vi "Send_Duration(SubVI).vi"(9 "error in (no error)":errorcluster, 10 "VISA resource name":refnum<visa-resource-name>, 11 "Set High1 Time":i16) -> (0 "error out":errorcluster, 1 "ASCII string":string[](array[string]), 2 "High1 Time(ns)":dbl, 3 "Digital Outputs":bool[](array[boolean]), 5 "VISA resource name out":refnum<visa-resource-name>, 8 "In Range?":bool)   [LabVIEW 2022 SP3]
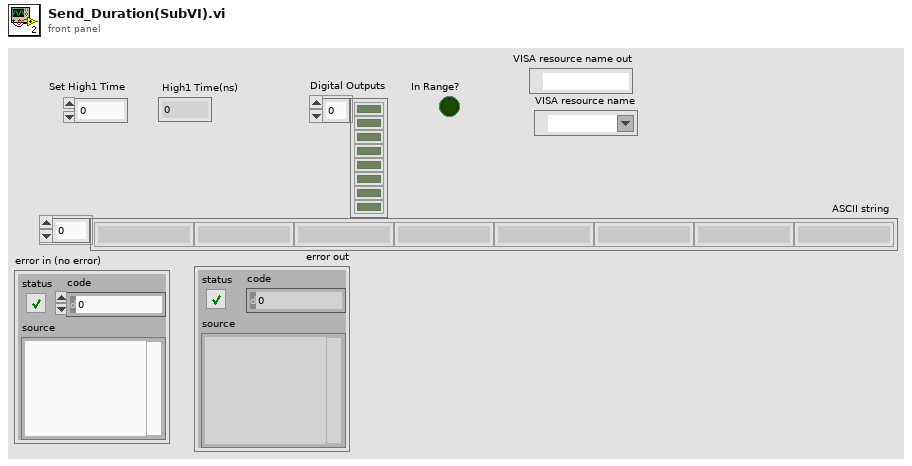
[diagram p1: front panel]
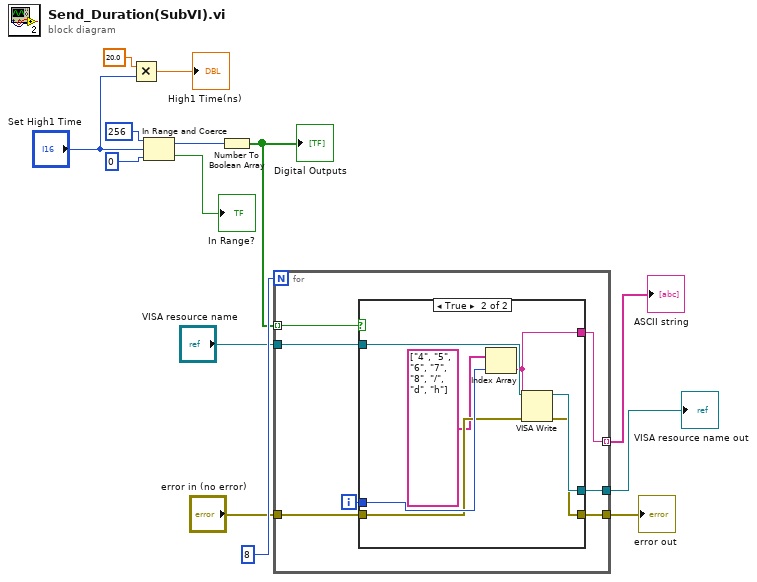
[diagram p0: block diagram]
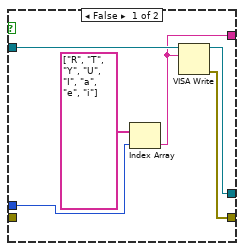
[diagram p2: hidden frame]
diagram:
  n1 = Multiply(x=20.0, y="Set High1 Time") -> (x*y=→"High1 Time(ns)":dbl)
  n2 = In Range and Coerce(upper limit=i16 256, x="Set High1 Time", lower limit=i8 0) -> (coerced(x)=w8:i16, In Range?=→"In Range?":bool)
  n3 = Number To Boolean Array(number=w8) -> (Boolean array=w9:bool[])
  "Digital Outputs" <- w9
  n4 = for {
    N: 8 -> [_]
    tunnel: w9 -> [w21] mode=indexing
    tunnel: [w19] -> w11 mode=indexing
    tunnel: "VISA resource name" -> [w18]
    tunnel: [w17] -> w3
    tunnel: [w16] -> w2
    tunnel: "error in (no error)" -> [w15]
    i -> [w20]
    n5 = case shown="True" w21 {
      tunnel: w20 -> [w27 w34]
      tunnel: [w25 w32] -> w19
      tunnel: w18 -> [w26 w33]
      tunnel: [w24 w31] -> w17
      tunnel: [w23 w30] -> w16
      tunnel: w15 -> [_ w29]
      frame False {
        n6 = Index Array(array=string[] ["R", "T", "Y", "U", "I", "a", "e", "i"] ("ASCII LOW"), index=w27) -> (element=w25:string)
        n7 = VISA Write(VISA resource name=w26, write buffer=w25) -> (VISA resource name out=w24:refnum<visa-resource-name>, error out=w23:errorcluster)  [unwired: 1 in, 1 out]
      }
      frame True {
        n8 = Index Array(array=string[] ["4", "5", "6", "7", "8", "/", "d", "h"] ("ASCII HIGH"), index=w34) -> (element=w32:string)
        n9 = VISA Write(VISA resource name=w33, write buffer=w32, error in (no error)=w29) -> (VISA resource name out=w31:refnum<visa-resource-name>, error out=w30:errorcluster)  [unwired: 1 out]
      }
    }
  }
  "ASCII string" <- w11
  "VISA resource name out" <- w3
  "error out" <- w2
